vi "Boolean and Compression Functions.vi"() -> ()   [LabVIEW 2022 SP3]
panel:
  out "s? t:f":dbl
  in  "f":dbl
  in  "t":dbl
  in  "Boolean 8":bool
  out "coerced(x)":dbl
  out "Boolean 7":bool
  in  "x":dbl
  out "Min":dbl
  out "Max":dbl
  in  "Numeric 2":dbl
  in  "Numeric":dbl
  out "Boolean 6":bool
  in  "Boolean 5":bool
  in  "Boolean 4":bool
  out "Boolean 3":bool
  in  "Boolean 2":bool
  in  "Boolean":bool
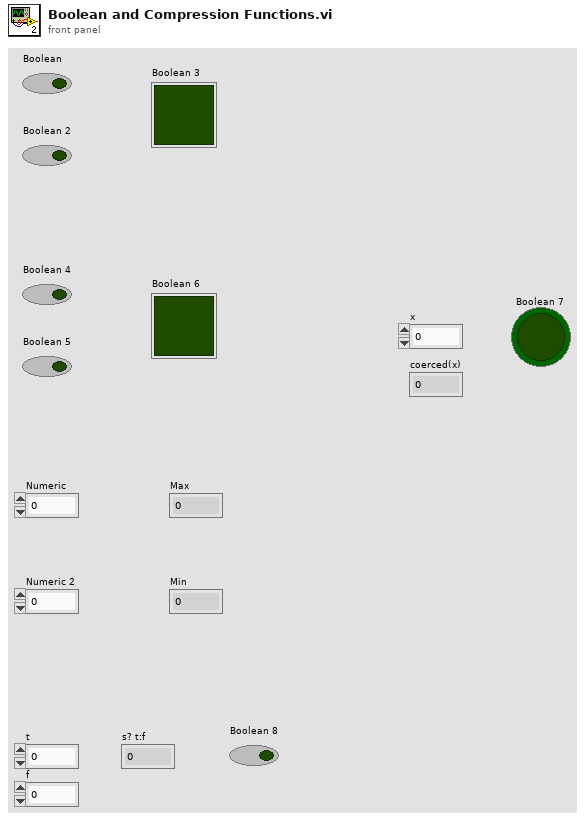
[diagram p1: front panel]
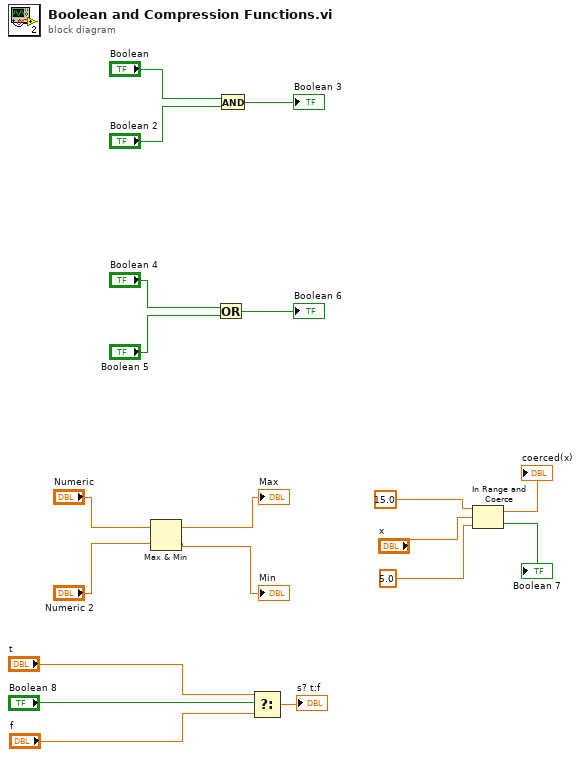
[diagram p0: block diagram]
diagram:
  n1 = Max & Min(x="Numeric", y="Numeric 2") -> (max(x,y)=→"Max":dbl, min(x,y)=→"Min":dbl)
  n2 = Or(x="Boolean 4", y="Boolean 5") -> (x .or. y?=→"Boolean 6":bool)
  n3 = And(x="Boolean", y="Boolean 2") -> (x .and. y?=→"Boolean 3":bool)
  n4 = Select(t="t", s="Boolean 8", f="f") -> (s? t:f=→"s? t:f":dbl)
  n5 = In Range and Coerce(upper limit=15.0, x="x", lower limit=5.0) -> (coerced(x)=→"coerced(x)":dbl, In Range?=→"Boolean 7":bool)
